vi "SEQ Obtain.vi"(8 "error in":errorcluster) -> (0 "error out":errorcluster, 3 "queue out":refnum<queue>)   [LabVIEW 2019, in "Image.lvlib"]
uses:
  Image.lvlib
  SEQ Data.ctl
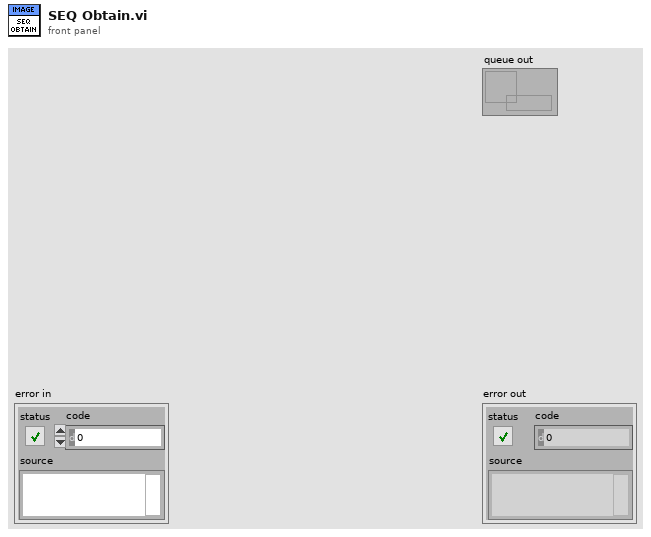
[diagram p1: front panel]
types:
  T1 = typedef "Image.lvlib/SEQ Data.ctl" = cluster{"Acquire Done?":bool, "Focus Done?":bool, "Align Done?":bool, "No Position Match?":bool, "Best Wheel Position":string, "Match Done?":bool, "Match Score":dbl, "Focus Score":dbl, "Match Position":cluster{"x":sgl, "y":sgl}, "Flower Position":i32[]}
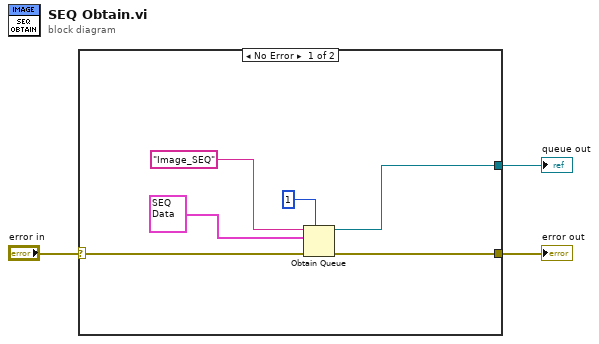
[diagram p0: block diagram]
diagram:
  n1 = case shown="No Error" "error in" {
    selector: "error in" -> [w9 w10]
    tunnel: [w8 w10] -> w2
    tunnel: [w4 _] -> w1
    frame No Error {
      n2 = Obtain Queue(max queue size (-1, unlimited)=1, name (unnamed)="Image_SEQ", element data type=T1 {"Acquire Done?"=FALSE, "Focus Done?"=FALSE, "Align Done?"=FALSE, "No Position Match?"=FALSE, "Best Wheel Position"="", "Match Done?"=FALSE, "Match Score"=0.0, "Focus Score"=0.0, "Match Position"={"x"=0.0, "y"=0.0}, "Flower Position"=[]} ("Cluster"), error in (no error)=w9) -> (queue out=w4:refnum<queue>, error out=w8:errorcluster)  [unwired: 1 in, 1 out]
    }
    frame Error {
    }
  }
  "error out" <- w2
  "queue out" <- w1
